vi "Get New Records for Posting.vi"(4 "error IN":errorcluster) -> (0 "error out":errorcluster, 2 "shots recordset":variant[][](array[variant]), 3 "expt recordset":variant[][](array[variant]))   [LabVIEW 2010]
uses:
  <vilib>/addons/database/NI_Database_API.lvlib
  <vilib>/addons/database/Connection.llb/DB Tools Open Connec (Path).vi
  <vilib>/addons/database/Connection.llb/Conn Execute.vi
  <vilib>/addons/database/Recordset.llb/Rec Destroy - Connection.vi
  <vilib>/addons/database/Recordset.llb/Rec Save Recordset To File (R).vi
  <vilib>/addons/database/Recordset.llb/Rec Fetch Recordset Data (R).vi
panel:
  in  "expt seed":i16=2208
  in  "shot seed":i16=4396
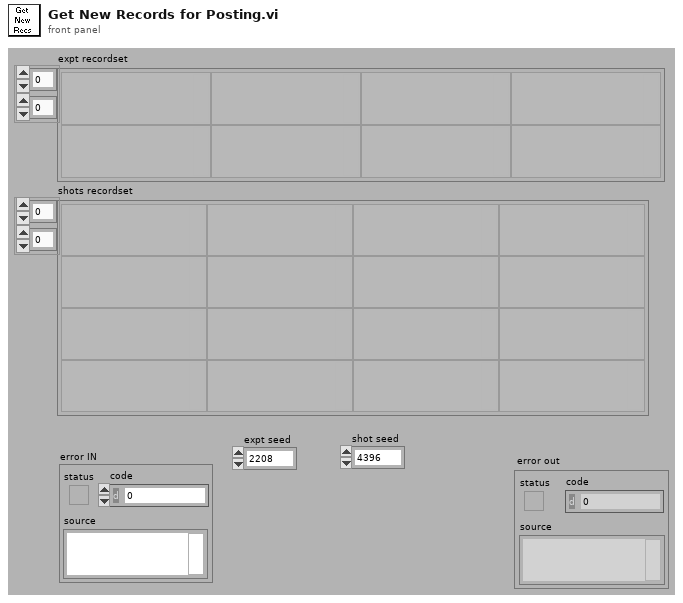
[diagram p1: front panel]
types:
  T1 = typedef "NI_Database_API.lvlib/Conn ObjectReference.ctl" = refnum<k1>
  T2 = typedef "NI_Database_API.lvlib/Rec ObjectReference.ctl" = refnum<k1>
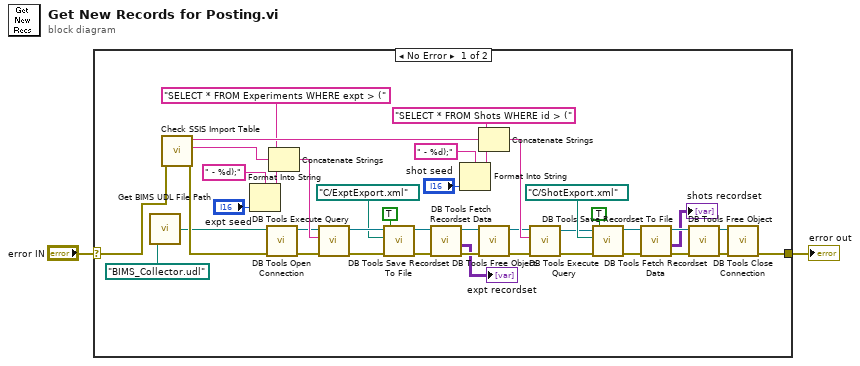
[diagram p0: block diagram]
diagram:
  n1 = case shown="No Error" "error IN" {
    selector: "error IN" -> [w31 w44]
    tunnel: [w30 w44] -> w1
    frame No Error {
      n2 = call "Get BIMS UDL File Path.vi"("UDL file name"=path "BIMS_Collector.udl" ("connectString")) -> ("Full UDL file path"=w29:path)
      n3 = call "Check SSIS Import Table.vi"("error IN"=w31) -> ("error OUT"=w41:errorcluster, "max expt rec"=w43:string, "max shot id rec"=w42:string)  [unwired: 1 in, 7 out]
      n4 = Format Into String(format string=" - %d);" ("message"), "expt seed") -> (resulting string=w22:string)  [unwired: 2 in, 1 out]
      n5 = call-poly <vilib>:"DB Tools Open Connection.vi"("error in (no error)"=w41, "connection information"=w29) -> ("error out"=w33:errorcluster, "connection reference"=w32:T1)  [unwired: 3 in, 3 out]
      n6 = Concatenate Strings("SELECT * FROM Experiments WHERE expt > (" ("message"), w43, w22) -> (w35:string)
      n7 = call-poly <vilib>:"DB Tools Execute Query.vi"("error in (no error)"=w33, "SQL query"=w35, "connection reference"=w32) -> ("error out"=w20:errorcluster, "recordset reference"=w21:T2)  [unwired: 1 in, 4 out]
      n8 = call-poly <vilib>:"DB Tools Save Recordset To File.vi"("overwrite? (F)"=TRUE ("overwrite? (f)"), "error in (no error)"=w20, "file name"=path "C:/ExptExport.xml" ("connectString"), "recordset reference"=w21) -> ("error out"=w3:errorcluster, "recordset reference out"=w4:T2)  [unwired: 1 in, 3 out]
      n9 = call-poly <vilib>:"DB Tools Fetch Recordset Data.vi"("error in (no error)"=w3, "recordset reference"=w4) -> ("error out"=w8:errorcluster, "recordset data"=→"expt recordset":variant[][], "recordset reference out"=w9:T2)  [unwired: 3 out]
      n10 = Format Into String(format string=" - %d);" ("message"), "shot seed") -> (resulting string=w25:string)  [unwired: 2 in, 1 out]
      n11 = Concatenate Strings("SELECT * FROM Shots WHERE id > (" ("message"), w42, w25) -> (w40:string)
      n12 = call-poly <vilib>:"DB Tools Free Object.vi"("error in (no error)"=w8, "recordset reference"=w9) -> ("error out"=w14:errorcluster, "connection reference"=w37:T1)  [unwired: 8 out]
      n13 = call-poly <vilib>:"DB Tools Execute Query.vi"("error in (no error)"=w14, "SQL query"=w40, "connection reference"=w37) -> ("error out"=w13:errorcluster, "recordset reference"=w15:T2)  [unwired: 1 in, 4 out]
      n14 = call-poly <vilib>:"DB Tools Save Recordset To File.vi"("overwrite? (F)"=TRUE ("overwrite? (f)"), "error in (no error)"=w13, "file name"=path "C:/ShotExport.xml" ("connectString"), "recordset reference"=w15) -> ("error out"=w6:errorcluster, "recordset reference out"=w5:T2)  [unwired: 1 in, 3 out]
      n15 = call-poly <vilib>:"DB Tools Fetch Recordset Data.vi"("error in (no error)"=w6, "recordset reference"=w5) -> ("error out"=w12:errorcluster, "recordset data"=→"shots recordset":variant[][], "recordset reference out"=w11:T2)  [unwired: 3 out]
      n16 = call-poly <vilib>:"DB Tools Free Object.vi"("error in (no error)"=w12, "recordset reference"=w11) -> ("error out"=w39:errorcluster, "connection reference"=w38:T1)  [unwired: 8 out]
      n17 = call <vilib>:"DB Tools Close Connection.vi"("error in (no error)"=w39, "connection reference"=w38) -> ("error out"=w30:errorcluster)  [unwired: 5 out]
    }
    frame Error {
    }
  }
  "error out" <- w1
